vi "Transition DSP402.vi"(1 "New state":T1, 2 "Old state":T1) -> (0 "Transition":i32)   [LabVIEW 2026, in "canopen_.lvlib" / "DSP402.lvclass"]
uses:
  DSP402.lvclass
  DSP402.lvclass/DSP402.ctl
  DriveState.ctl
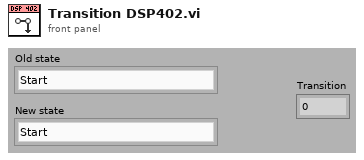
[diagram p1: front panel]
types:
  T1 = typedef "canopen_.lvlib/DSP402.lvclass/DriveState.ctl" = enum16{"Start", "Not ready to switch on", "Switch on disabled", "Ready to switch on", "Switched on", "Operation enable", "Fault reaction active", "Fault", "Quick stop active"}
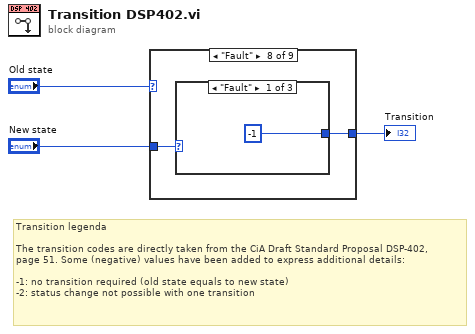
[diagram p0: block diagram]
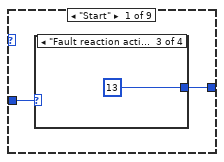
[diagram p2: hidden frame]
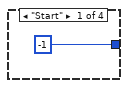
[diagram p3: hidden frame]
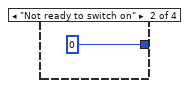
[diagram p4: hidden frame]
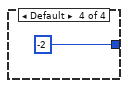
[diagram p5: hidden frame]
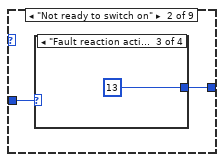
[diagram p6: hidden frame]
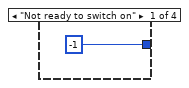
[diagram p7: hidden frame]
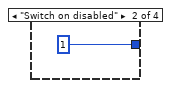
[diagram p8: hidden frame]
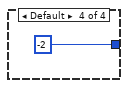
[diagram p9: hidden frame]
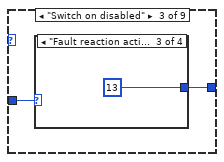
[diagram p10: hidden frame]
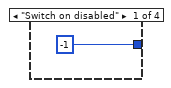
[diagram p11: hidden frame]
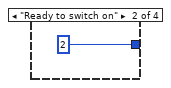
[diagram p12: hidden frame]
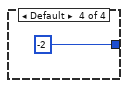
[diagram p13: hidden frame]
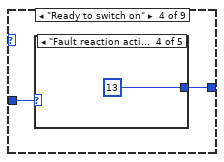
[diagram p14: hidden frame]
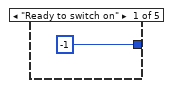
[diagram p15: hidden frame]
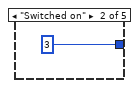
[diagram p16: hidden frame]
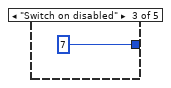
[diagram p17: hidden frame]
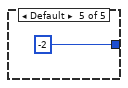
[diagram p18: hidden frame]
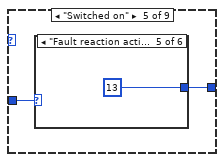
[diagram p19: hidden frame]
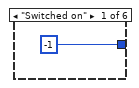
[diagram p20: hidden frame]
diagram:
  # "Transition legenda\n\nThe transition codes are directly taken from the CiA Draft Standard Proposal DSP-402,\npage 51. Some (negative) values have been added to express additional details:\n\n-1: no transition required (old state equals to new state)\n-2: status change not possible with one transition"
  n1 = case shown="\"Fault\"" "Old state" {
    tunnel: "New state" -> [w5 w11 w17 w23 w30 w38 w47 w52 w57]
    tunnel: [w4 w10 w16 w22 w29 w37 w46 w51 w56] -> w2
    frame "Start" {
      n2 = case shown="\"Fault reaction active\"" w5 {
        tunnel: [-1 0 13 -2] -> w4
        frame "Start" {
        }
        frame "Not ready to switch on" {
        }
        frame "Fault reaction active" {
        }
        frame Default {
        }
      }
    }
    frame "Not ready to switch on" {
      n3 = case shown="\"Fault reaction active\"" w11 {
        tunnel: [-1 1 13 -2] -> w10
        frame "Not ready to switch on" {
        }
        frame "Switch on disabled" {
        }
        frame "Fault reaction active" {
        }
        frame Default {
        }
      }
    }
    frame "Switch on disabled" {
      n4 = case shown="\"Fault reaction active\"" w17 {
        tunnel: [-1 2 13 -2] -> w16
        frame "Switch on disabled" {
        }
        frame "Ready to switch on" {
        }
        frame "Fault reaction active" {
        }
        frame Default {
        }
      }
    }
    frame "Ready to switch on" {
      n5 = case shown="\"Fault reaction active\"" w23 {
        tunnel: [-1 3 7 13 -2] -> w22
        frame "Ready to switch on" {
        }
        frame "Switched on" {
        }
        frame "Switch on disabled" {
        }
        frame "Fault reaction active" {
        }
        frame Default {
        }
      }
    }
    frame "Switched on" {
      n6 = case shown="\"Fault reaction active\"" w30 {
        tunnel: [-1 4 6 10 13 -2] -> w29
        frame "Switched on" {
        }
        frame "Operation enable" {
        }
        frame "Ready to switch on" {
        }
        frame "Switch on disabled" {
        }
        frame "Fault reaction active" {
        }
        frame Default {
        }
      }
    }
    frame "Operation enable" {
      n7 = case shown="\"Fault reaction active\"" w38 {
        tunnel: [-1 11 5 8 9 13 -2] -> w37
        frame "Operation enable" {
        }
        frame "Quick stop active" {
        }
        frame "Switched on" {
        }
        frame "Ready to switch on" {
        }
        frame "Switch on disabled" {
        }
        frame "Fault reaction active" {
        }
        frame Default {
        }
      }
    }
    frame "Fault reaction active" {
      n8 = case shown="Default" w47 {
        tunnel: [-1 14 -2] -> w46
        frame "Fault reaction active" {
        }
        frame "Fault" {
        }
        frame Default {
        }
      }
    }
    frame "Fault" {
      n9 = case shown="\"Fault\"" w52 {
        tunnel: [-1 15 -2] -> w51
        frame "Fault" {
        }
        frame "Switch on disabled" {
        }
        frame Default {
        }
      }
    }
    frame "Quick stop active" {
      n10 = case shown="Default" w57 {
        tunnel: [-1 16 12 13 -2] -> w56
        frame "Quick stop active" {
        }
        frame "Operation enable" {
        }
        frame "Switch on disabled" {
        }
        frame "Fault reaction active" {
        }
        frame Default {
        }
      }
    }
  }
  "Transition" <- w2
